vi "Search and Filter Properties.vi"(7 "Search Keys":string[](array[string]), 9 "Values In":string[](array[string]), 10 "Types In":T1[](array[typedef]), 11 "Keys In":string[](array[string])) -> (0 "Filtered Values":string[](array[string]), 1 "Values":string[](array[string]), 2 "Types":T1[](array[typedef]), 3 "Keys":string[](array[string]), 4 "Item Found":bool[](array[boolean]), 5 "Filtered Types":T1[](array[typedef]))   [LabVIEW 2020, in "JSON.lvlib"]
doc: "This VI is meant to follow <b>Parse Object Properties</b> and aids in pulling out specific properties by name. For each specified key to search for, a boolean value is returned determining if the key was present, the type of the matched value, and the string representation of the value. The 3 input arrays from Parse Object Properties are passed as-is to the output arrays and filtered values are not removed."
uses:
  JSON.lvlib
  JSON Item Type.ctl
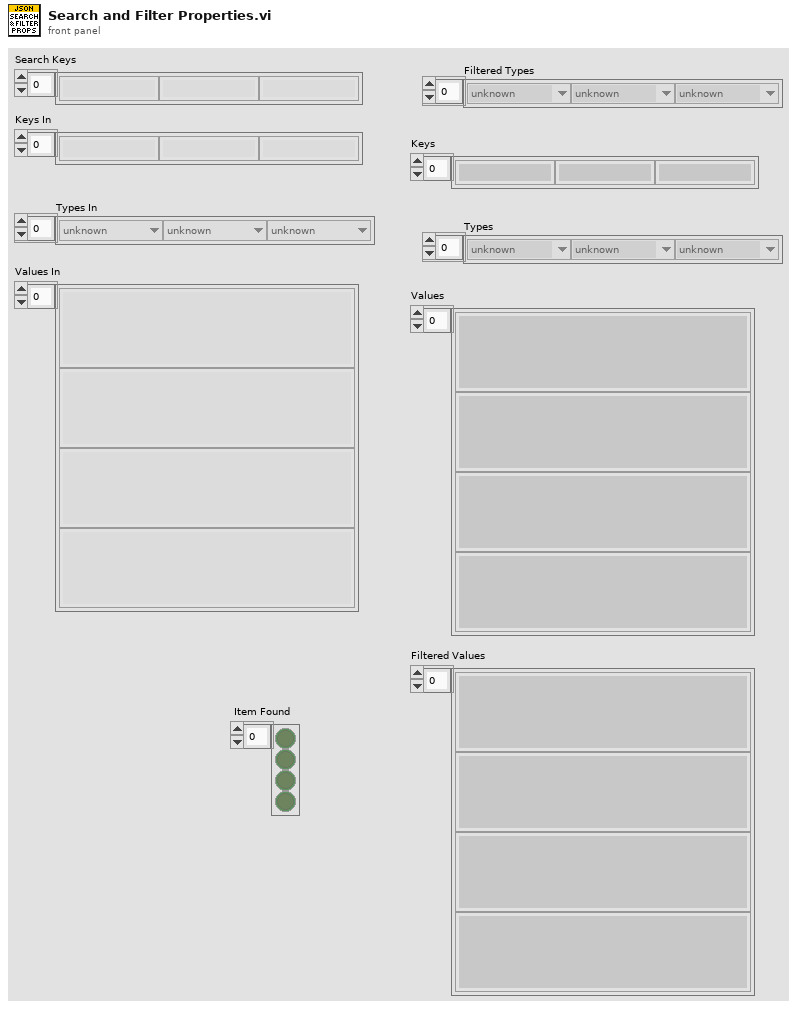
[diagram p1: front panel]
types:
  T1 = typedef "JSON.lvlib/JSON Item Type.ctl" = enum16{"unknown", "null", "Array", "Object", "String", "Number", "Boolean"}
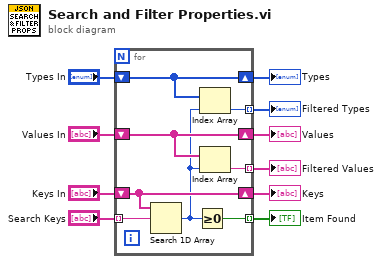
[diagram p0: block diagram]
diagram:
  n1 = for {
    shift-right: [w17] -> w2
    shift-left: "Keys In" -> [w17]
    shift-right: [w16] -> w3
    shift-left: "Values In" -> [w16]
    tunnel: "Search Keys" -> [w18] mode=indexing
    tunnel: [w15] -> w7 mode=indexing
    tunnel: [w14] -> w6 mode=indexing
    shift-right: [w12] -> w4
    shift-left: "Types In" -> [w12]
    tunnel: [w11] -> w1 mode=indexing
    n2 = Search 1D Array(1D array=w17, element=w18) -> (index of element=w13:i32)  [unwired: 1 in]
    n3 = Greater Or Equal To 0?(x=w13) -> (x >= 0?=w14:bool)
    n4 = Index Array(array=w12, index=w13) -> (element=w11:T1)
    n5 = Index Array(array=w16, index=w13) -> (element=w15:string)
  }
  "Keys" <- w2
  "Values" <- w3
  "Item Found" <- w6
  "Filtered Values" <- w7
  "Types" <- w4
  "Filtered Types" <- w1
